vi "VoltageOutputSetEnabled.vi"(0 "error in (no error)":errorcluster, 2 "Enabled":bool, 3 "Device In":u64) -> (7 "error out":errorcluster, 10 "Device Out":u64)   [LabVIEW 2012, in "Phidget Voltage Output.lvlib"]
doc: "${Enabled:Header}"
uses:
  <instrlib>/Phidgets/Phidget Voltage Output/Phidget Voltage Output.lvlib
  <instrlib>/Phidgets/Phidget Common/Phidget Common.lvlib
  phidget22.dll
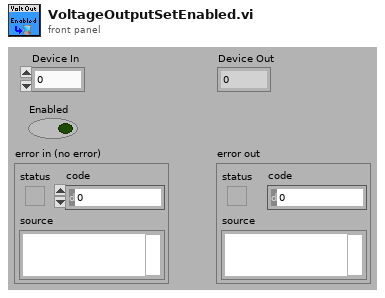
[diagram p1: front panel]
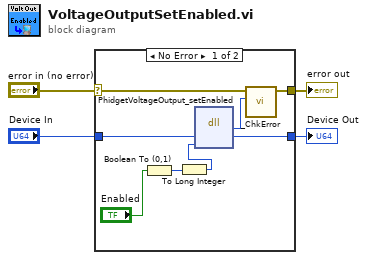
[diagram p0: block diagram]
diagram:
  n1 = case shown="No Error" "error in (no error)" {
    selector: "error in (no error)" -> [w10 w14]
    tunnel: [w9 w14] -> w3
    tunnel: "Device In" -> [w12 w13]
    tunnel: [w11 w13] -> w1
    frame No Error {
      n2 = Boolean To (0,1)(Boolean="Enabled") -> (0, 1=w6:i16)
      n3 = To Long Integer(number=w6) -> (32bit integer=w5:i32)
      n4 = dll-call lib="phidget22.*" fn="PhidgetVoltageOutput_setEnabled"("phid"=w12, "interval"=w5) -> ("return type"=w8:i32, "phid"=w11:u64)  [unwired: 4 in, 2 out]
      n5 = call <instrlib>:"_ChkError.vi"("Return Code"=w8, "error in (no error)"=w10) -> ("error out"=w9:errorcluster)  [unwired: 9 in]
    }
    frame Error {
    }
  }
  "error out" <- w3
  "Device Out" <- w1
